vi "Ablasión_2024.vi"() -> ()   [LabVIEW 2021]
uses:
  <vilib>/DAQmx/write.llb/DAQmx Write (Digital Bool 1Line 1Point).vi
  <vilib>/Utility/file.llb/Read Delimited Spreadsheet (DBL).vi
  <vilib>/DAQmx/miscellaneous.llb/DAQmx Fill In Error Info.vi
panel:
  in  "Apagar":bool
  out "Estado del Láser":bool
  in  "Iniciar":bool
  in  "Posición Relativa":dbl[](array[numeric])
  in  "Ir origen":bool
  in  "N. Origen":bool
  in  "Mover":bool
  in  "Ablasión":bool
  in  "Nombre para el CSV":string
  in  "Config. Láser":refnum<k21>
  in  "Path CSV":path
  in  "Path Dibujador":path
  in  "Ancho":string
  in  "Alto":string
  in  "Tamaño Pixel":string
  in  "Detener":bool
  out "Ejes":dbl=2.0
  out "CU ID":i32=1 min=1 max=20
  # "ABLACIÓN LÁSER"
  # "Movimiento de Motores"
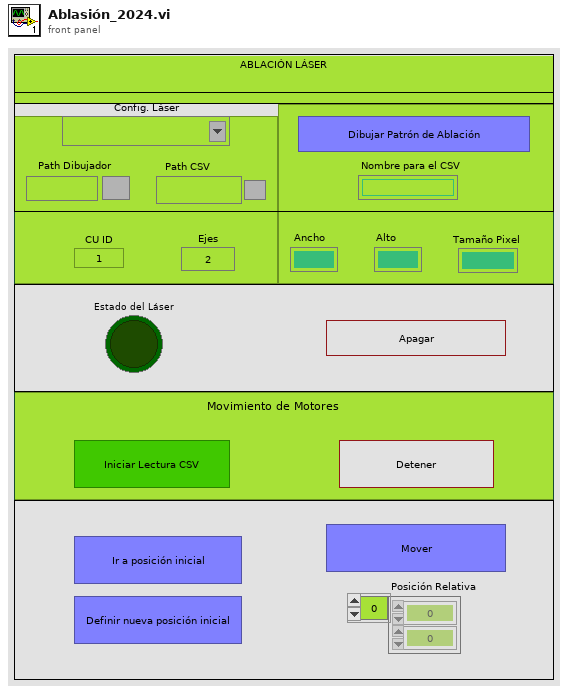
[diagram p1: front panel]
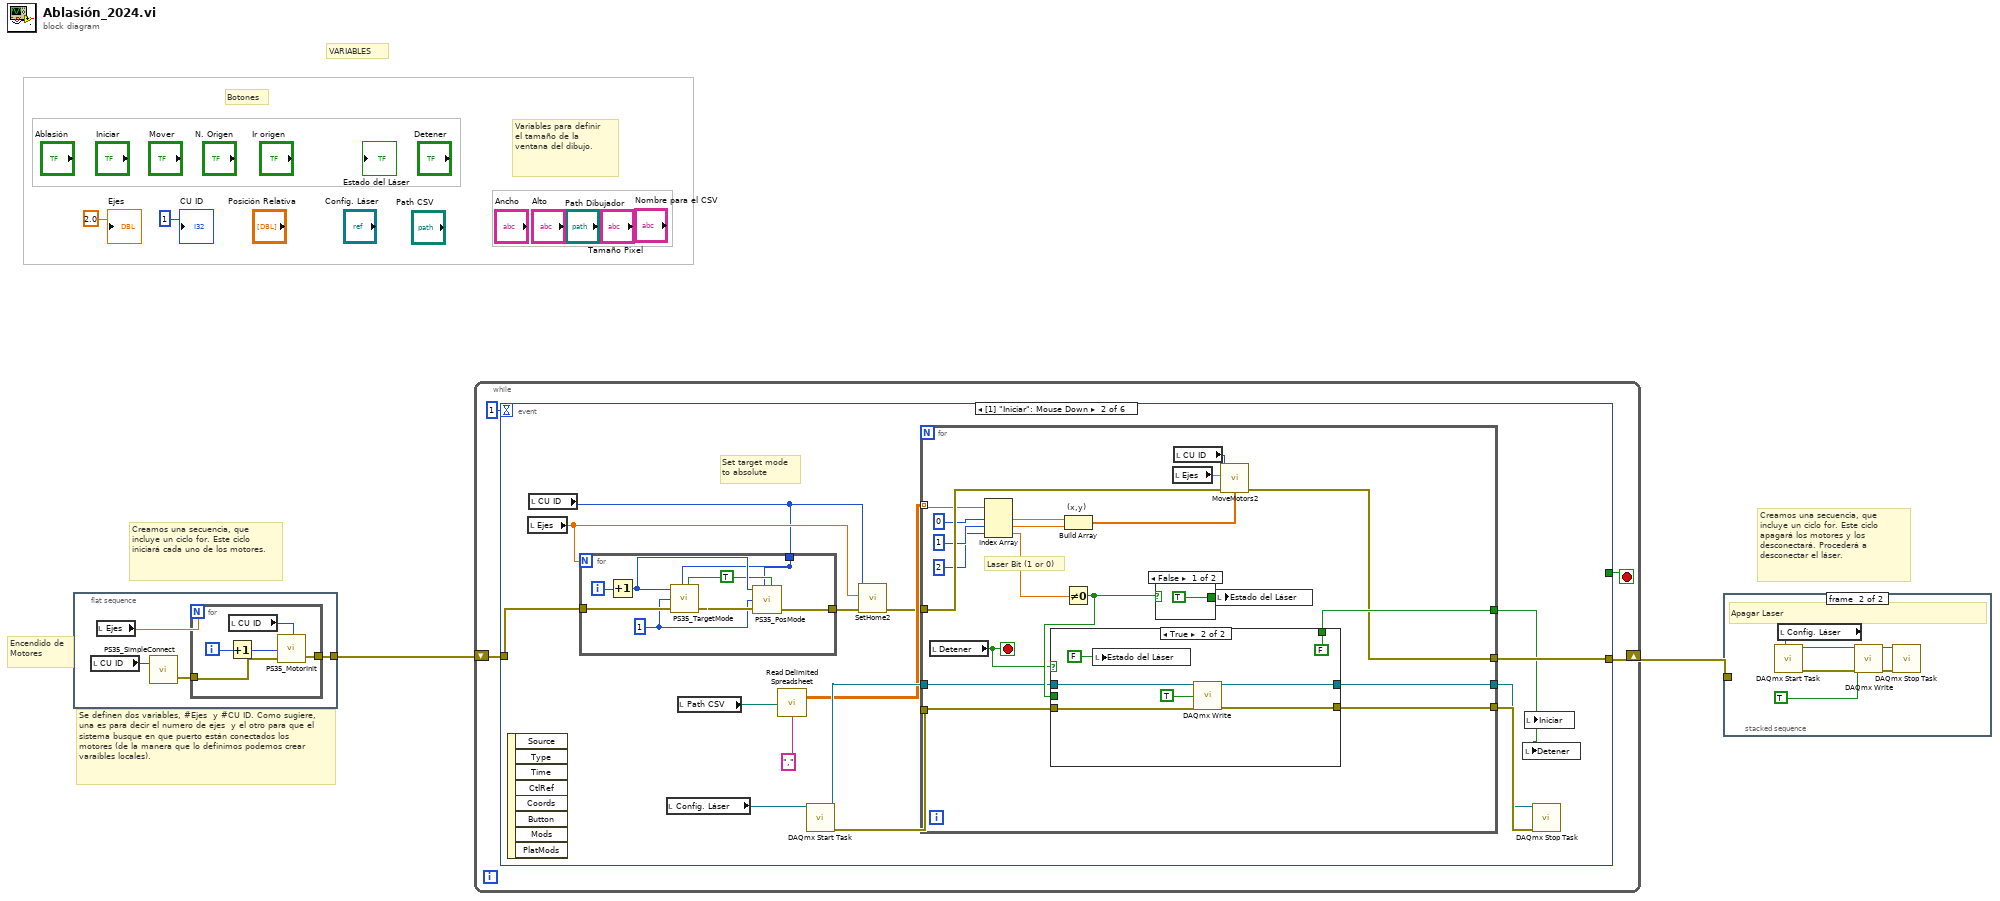
[diagram p0: block diagram]
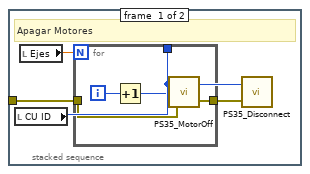
[diagram p2: hidden frame]
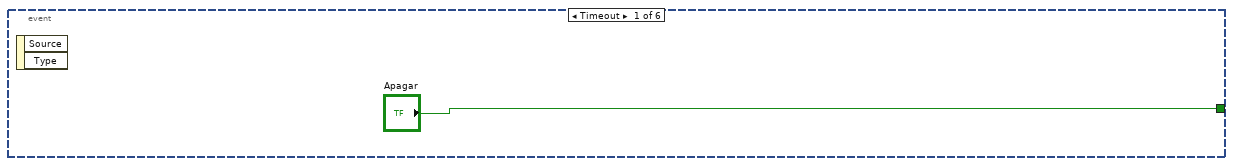
[diagram p3: hidden frame]
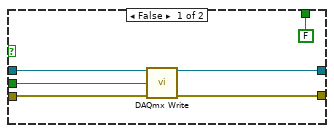
[diagram p4: hidden frame]
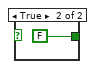
[diagram p5: hidden frame]
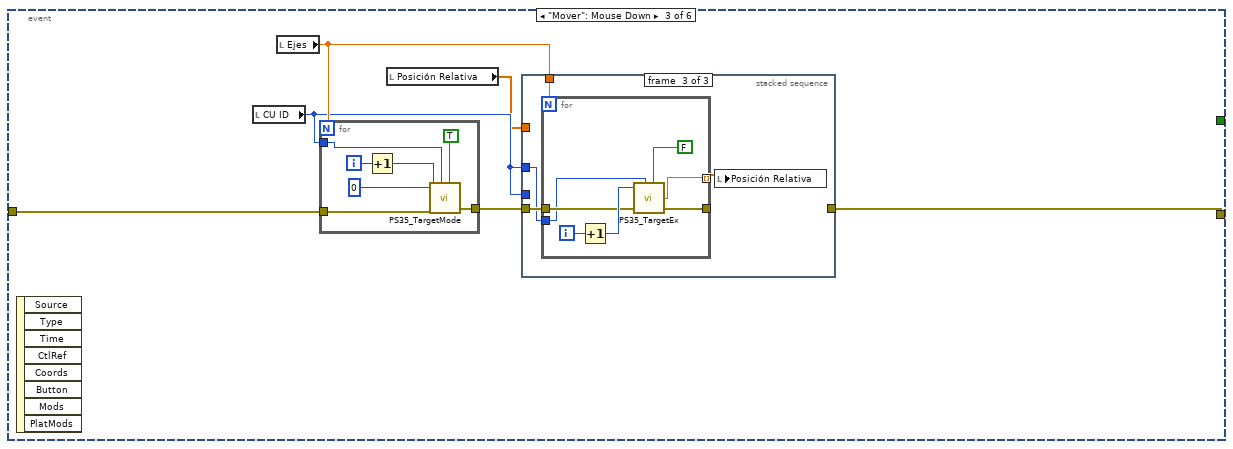
[diagram p6: hidden frame]
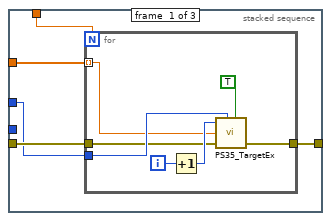
[diagram p7: hidden frame]
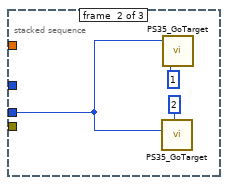
[diagram p8: hidden frame]
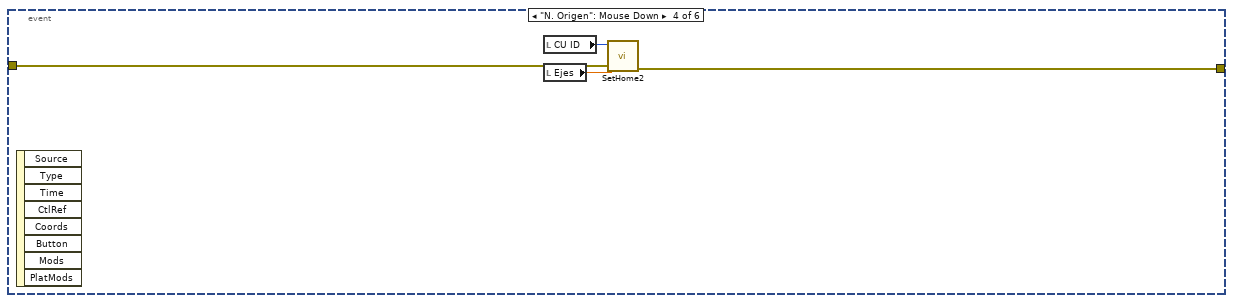
[diagram p9: hidden frame]
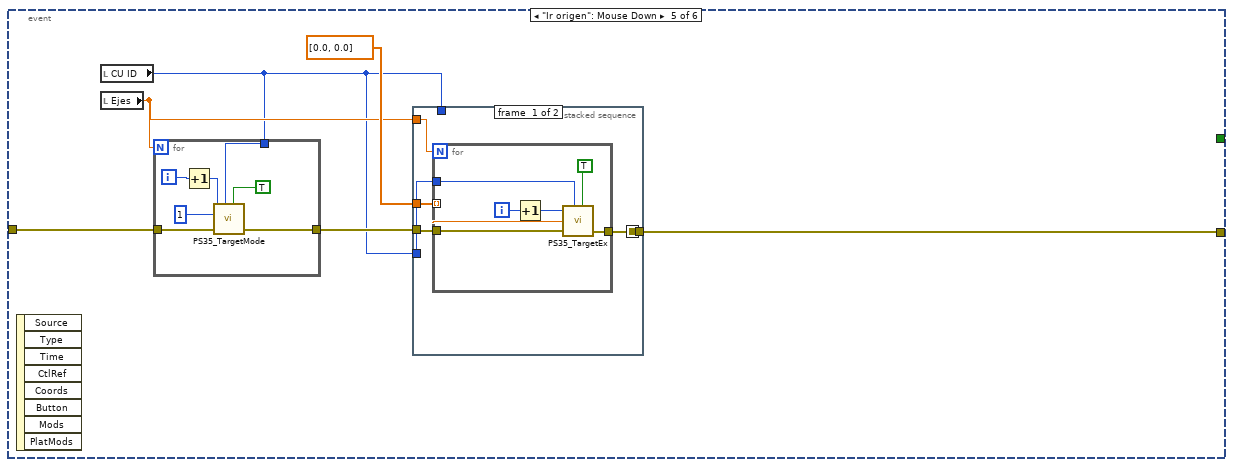
[diagram p10: hidden frame]
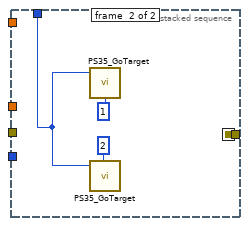
[diagram p11: hidden frame]
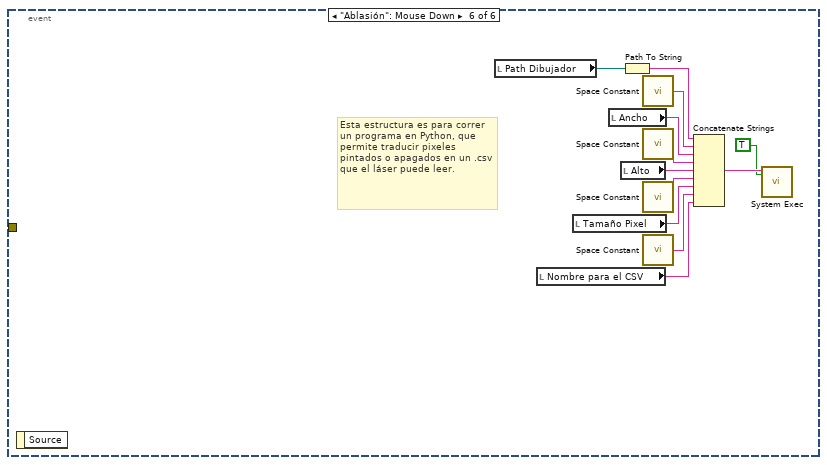
[diagram p12: hidden frame]
diagram:
  # "VARIABLES"
  # "Botones"
  # "Variables para definir el tamaño de la ventana del dibujo."
  # "Creamos una secuencia, que incluye un ciclo for. Este ciclo apagará los motores y los desconectará. Procederá a desconectar el láser."
  # "Se definen dos variables, #Ejes  y #CU ID. Como sugiere, una es para decir el numero de ejes  y el otro para que el sistema busque en que puerto están conectados los motores (de la manera que lo definimos podemos crear varaibles locales)."
  # "Creamos una secuencia, que incluye un ciclo for. Este ciclo iniciará cada uno de los motores."
  # "Encendido de Motores"
  n1 = flat-sequence {
    tunnel: [w7] -> w2
    frame #0 {
      n2 = local read "CU ID"() -> (w5:i32)
      n3 = local read "Ejes"() -> (w6:dbl)
      n4 = call "PS35_SimpleConnect.vi"("Control unit ID"=w5) -> ("error out"=w8:errorcluster)  [unwired: 3 in]
      n5 = for {
        N: w6 -> [_]
        tunnel: w8 -> [w11]
        tunnel: [w10] -> w7
        i -> [w13]
        n6 = Increment(x=w13) -> (x+1=w12:i32)
        n7 = local read "CU ID"() -> (w9:i32)
        n8 = call "PS35_MotorInit.vi"("error in (no error)"=w11, "Axis number"=w12, "Control unit ID"=w9) -> ("error out"=w10:errorcluster)  [unwired: 1 in]
      }
    }
  }
  n9 = while {
    shift-right: [w16] -> w1
    shift-left: w2 -> [w17]
    stop <- w14 stop-if-true
    n10 = event shown="[1] \"Iniciar\": Mouse Down" {
      selector: _ -> [_ _ _ _ _ _]
      dyn-events: _ -> [_ _ _ _ _ _]
      timeout: 1 -> [_ _ _ _ _ _]
      tunnel: w17 -> [_ w27 w78 w117 w125 _]
      tunnel: [_ w26 w77 w116 w120 _] -> w16
      tunnel: ["Apagar" _ _ _ _ _] -> w14
      event Timeout {
        n11 = event-data() -> ()  [unwired: 1 in, 2 out]
      }
      event "Iniciar": Mouse Down {
        # "Set target mode\nto absolute"
        n12 = event-data() -> ()  [unwired: 1 in, 8 out]
        n13 = local read "Ejes"() -> (w23:dbl)
        n14 = local read "CU ID"() -> (w22:i32)
        n15 = for {
          N: w23 -> [_]
          tunnel: [w38] -> w24
          tunnel: w27 -> [w41]
          tunnel: w22 -> [w34]
          i -> [w40]
          w37 = 1 ("Value-In")
          w35 = TRUE ("function")
          n16 = Increment(x=w40) -> (x+1=w36:i32)
          n17 = call "PS35_TargetMode.vi"("Axis number"=w36, "Control unit ID"=w34, "Value-In"=w37, "error in (no error)"=w41, "function"=w35) -> ("error out"=w39:errorcluster)  [unwired: 3 in, 1 out]
          n18 = call "PS35_PosMode.vi"("Axis number"=w36, "Control unit ID"=w34, "Value-In"=w37, "error in (no error)"=w39, "function"=w35) -> ("error out"=w38:errorcluster)  [unwired: 3 in, 1 out]
        }
        n19 = local read "Config. Láser"() -> (w21:refnum<k21>)
        n20 = local read "Path CSV"() -> (w20:path)
        n21 = call-poly <vilib>:"Read Delimited Spreadsheet.vi"("file path (dialog if empty)"=w20, "delimiter (\\t)"="," ("delimiter (\\t)")) -> ("all rows"=w29:dbl[][])  [unwired: 8 in, 5 out]
        n22 = call <vilib>:"DAQmx Start Task.vi"("task/channels in"=w21) -> ("task out"=w30:refnum<k21>, "error out"=w31:errorcluster)  [unwired: 13 in]
        n23 = call "SetHome2.vi"("error in (no error)"=w24, "N Ax"=w23, "CU ID"=w22) -> ("error out"=w25:errorcluster)  [unwired: 8 in]
        n24 = for {
          tunnel: w25 -> [w61]
          tunnel: w29 -> [w57] mode=indexing
          tunnel: w30 -> [w52]
          tunnel: w31 -> [w51]
          tunnel: [w50] -> w32
          tunnel: [w49] -> w33
          tunnel: [w48] -> w19
          tunnel: [w46] -> w26
          stop <- w42 stop-if-true
          # "Laser Bit (1 or 0)"
          n25 = local read "Detener"() -> (w42:bool)
          n26 = Index Array(array=w57, index #1=0 ("index"), index #2=1 ("index"), index #3=2 ("index")) -> (element #1=w56:dbl, element #2=w55:dbl, element #3=w54:dbl)
          n27 = Build Array "(x,y)"(w56, w55) -> (w47:dbl[])
          n28 = Not Equal To 0?(x=w54) -> (x != 0?=w53:bool)
          n29 = case shown="True" w42 {
            tunnel: w53 -> [w67 _]
            tunnel: w52 -> [w66 w71]
            tunnel: w51 -> [w65 w72]
            tunnel: [w64 w74] -> w50
            tunnel: [w63 w73] -> w49
            tunnel: [FALSE ("ABORT") FALSE ("ABORT")] -> w48
            frame False {
              n30 = call-poly <vilib>:"DAQmx Write.vi"("task/channels in"=w66, "data"=w67, "error in"=w65) -> ("task out"=w64:refnum<k21>, "error out"=w63:errorcluster)  [unwired: 10 in, 1 out]
            }
            frame True {
              n31 = local write "Estado del Láser"(FALSE ("Laser ON/OFF")) -> ()
              n32 = call-poly <vilib>:"DAQmx Write.vi"("task/channels in"=w71, "data"=TRUE, "error in"=w72) -> ("task out"=w74:refnum<k21>, "error out"=w73:errorcluster)  [unwired: 10 in, 1 out]
            }
          }
          n33 = case shown="False" w53 {
            tunnel: [TRUE FALSE] -> w43
            frame False {
            }
            frame True {
            }
          }
          n34 = local read "Ejes"() -> (w45:dbl)
          n35 = local read "CU ID"() -> (w44:i32)
          n36 = local write "Estado del Láser"(w43) -> ()
          n37 = call "MoveMotors2.vi"("error in (no error)"=w61, "Target"=w47, "N Ax"=w45, "CU ID"=w44) -> ("error out"=w46:errorcluster)  [unwired: 7 in]
        }
        n38 = local write "Detener"(w19) -> ()
        n39 = local write "Iniciar"(w19) -> ()
        n40 = call <vilib>:"DAQmx Stop Task.vi"("task/channels in"=w32, "error in"=w33) -> ()  [unwired: 12 in, 2 out]
      }
      event "Mover": Mouse Down {
        n41 = event-data() -> ()  [unwired: 1 in, 8 out]
        n42 = local read "CU ID"() -> (w81:i32)
        n43 = local read "Ejes"() -> (w82:dbl)
        n44 = for {
          N: w82 -> [_]
          tunnel: w81 -> [w114]
          tunnel: [w110] -> w79
          tunnel: w78 -> [w109]
          i -> [w115]
          n45 = Increment(x=w115) -> (x+1=w111:i32)
          n46 = call "PS35_TargetMode.vi"("Axis number"=w111, "Control unit ID"=w114, "Value-In"=0, "error in (no error)"=w109, "function"=TRUE) -> ("error out"=w110:errorcluster)  [unwired: 3 in, 1 out]
        }
        n47 = local read "Posición Relativa"() -> (w80:dbl[])
        n48 = stacked-sequence {
          tunnel: w79 -> [w87 _ w100]
          tunnel: w81 -> [w86 _ w98]
          tunnel: w82 -> [w85 _ w101]
          tunnel: w81 -> [_ w95 _]
          tunnel: [w84 _ _] -> w77
          tunnel: w80 -> [w83 _ _]
          frame #0 {
            n49 = for {
              N: w85 -> [_]
              tunnel: w86 -> [w93]
              tunnel: w87 -> [w90]
              tunnel: [w89] -> w84
              tunnel: w83 -> [w88] mode=indexing
              i -> [w94]
              n50 = Increment(x=w94) -> (x+1=w91:i32)
              n51 = call "PS35_TargetEx.vi"("Axis number"=w91, "Control unit ID"=w93, "dValue-In"=w88, "error in (no error)"=w90, "function"=TRUE) -> ("error out"=w89:errorcluster)  [unwired: 3 in, 1 out]
            }
          }
          frame #1 {
            n52 = call "PS35_GoTarget.vi"("Axis number"=2, "Control unit ID"=w95) -> ()  [unwired: 2 in, 1 out]
            n53 = call "PS35_GoTarget.vi"("Axis number"=1, "Control unit ID"=w95) -> ()  [unwired: 2 in, 1 out]
          }
          frame #2 {
            n54 = for {
              N: w101 -> [_]
              tunnel: [w105] -> _
              tunnel: w100 -> [w104]
              tunnel: [w103] -> w99 mode=indexing
              tunnel: w98 -> [w102]
              i -> [w108]
              n55 = Increment(x=w108) -> (x+1=w106:i32)
              n56 = call "PS35_TargetEx.vi"("Axis number"=w106, "Control unit ID"=w102, "error in (no error)"=w104, "function"=FALSE) -> ("dValue-Out"=w103:dbl, "error out"=w105:errorcluster)  [unwired: 4 in]
            }
            n57 = local write "Posición Relativa"(w99) -> ()
          }
        }
      }
      event "N. Origen": Mouse Down {
        n58 = event-data() -> ()  [unwired: 1 in, 8 out]
        n59 = local read "CU ID"() -> (w118:i32)
        n60 = local read "Ejes"() -> (w119:dbl)
        n61 = call "SetHome2.vi"("error in (no error)"=w117, "N Ax"=w119, "CU ID"=w118) -> ("error out"=w116:errorcluster)  [unwired: 8 in]
      }
      event "Ir origen": Mouse Down {
        n62 = event-data() -> ()  [unwired: 1 in, 8 out]
        n63 = local read "CU ID"() -> (w121:i32)
        n64 = local read "Ejes"() -> (w122:dbl)
        n65 = for {
          N: w122 -> [_]
          tunnel: [w148] -> w124
          tunnel: w125 -> [w143]
          tunnel: w121 -> [w142]
          i -> [w146]
          n66 = Increment(x=w146) -> (x+1=w145:i32)
          n67 = call "PS35_TargetMode.vi"("Axis number"=w145, "Control unit ID"=w142, "Value-In"=1, "error in (no error)"=w143, "function"=TRUE) -> ("error out"=w148:errorcluster)  [unwired: 3 in, 1 out]
        }
        n68 = stacked-sequence {
          seq-local: [w127 _] -> [_ w138]
          tunnel: w124 -> [w130 _]
          tunnel: w121 -> [w128 _]
          tunnel: w122 -> [w129 _]
          tunnel: dbl[] [0.0, 0.0] ("Target") -> [w126 _]
          tunnel: w121 -> [_ w141]
          tunnel: [_ w138] -> w120
          frame #0 {
            n69 = for {
              N: w129 -> [_]
              tunnel: [w134] -> w127
              tunnel: w130 -> [w133]
              tunnel: w128 -> [w132]
              tunnel: w126 -> [w131] mode=indexing
              i -> [w137]
              n70 = Increment(x=w137) -> (x+1=w135:i32)
              n71 = call "PS35_TargetEx.vi"("Axis number"=w135, "Control unit ID"=w132, "dValue-In"=w131, "error in (no error)"=w133, "function"=TRUE) -> ("error out"=w134:errorcluster)  [unwired: 3 in, 1 out]
            }
          }
          frame #1 {
            n72 = call "PS35_GoTarget.vi"("Axis number"=1, "Control unit ID"=w141) -> ()  [unwired: 2 in, 1 out]
            n73 = call "PS35_GoTarget.vi"("Axis number"=2, "Control unit ID"=w141) -> ()  [unwired: 2 in, 1 out]
          }
        }
      }
      event "Ablasión": Mouse Down {
        # "Esta estructura es para correr un programa en Python, que permite traducir pixeles pintados o apagados en un .csv que el láser puede leer."
        n74 = event-data() -> ()  [unwired: 1 in, 1 out]
        n75 = local read "Path Dibujador"() -> (w150:path)
        n76 = local read "Nombre para el CSV"() -> (w160:string)
        n77 = local read "Tamaño Pixel"() -> (w158:string)
        n78 = local read "Ancho"() -> (w154:string)
        n79 = local read "Alto"() -> (w156:string)
        n80 = Path To String(path=w150) -> (string=w152:string)
        n81 = call <vilib>:"Space Constant.vi"() -> ("String"=w153:string)
        n82 = call <vilib>:"Space Constant.vi"() -> ("String"=w155:string)
        n83 = call <vilib>:"Space Constant.vi"() -> ("String"=w157:string)
        n84 = call <vilib>:"Space Constant.vi"() -> ("String"=w159:string)
        n85 = Concatenate Strings(w152, w153, w154, w155, w156, w157, w158, w159, w160) -> (w151:string)
        n86 = call <vilib>:"System Exec.vi"("wait until completion? (T)"=TRUE, "command line"=w151) -> ()  [unwired: 6 in, 4 out]
      }
    }
  }
  n87 = stacked-sequence {
    tunnel: w1 -> [w161 _]
    frame #0 {
      # "Apagar Motores"
      n88 = local read "CU ID"() -> (w163:i32)
      n89 = local read "Ejes"() -> (w164:dbl)
      n90 = for {
        N: w164 -> [_]
        tunnel: w163 -> [w168]
        tunnel: w161 -> [w167]
        tunnel: [w166] -> w162
        i -> [w169]
        n91 = Increment(x=w169) -> (x+1=w165:i32)
        n92 = call "PS35_MotorOff.vi"("error in (no error)"=w167, "Axis number"=w165, "Control unit ID"=w168) -> ("error out"=w166:errorcluster)  [unwired: 1 in]
      }
      n93 = call "PS35_Disconnect.vi"("error in (no error)"=w162, "Control unit ID"=w163) -> ()  [unwired: 1 in, 1 out]
    }
    frame #1 {
      # "Apagar Laser"
      n94 = local read "Config. Láser"() -> (w170:refnum<k21>)
      n95 = call <vilib>:"DAQmx Start Task.vi"("task/channels in"=w170) -> ("task out"=w174:refnum<k21>, "error out"=w175:errorcluster)  [unwired: 13 in]
      n96 = call-poly <vilib>:"DAQmx Write.vi"("task/channels in"=w174, "data"=TRUE, "error in"=w175) -> ("task out"=w171:refnum<k21>, "error out"=w172:errorcluster)  [unwired: 10 in, 1 out]
      n97 = call <vilib>:"DAQmx Stop Task.vi"("task/channels in"=w171, "error in"=w172) -> ()  [unwired: 12 in, 2 out]
    }
  }
  "CU ID" <- 1 ("CU ID")
  "Ejes" <- 2.0 ("N Ax")
